vi "判断调焦 - 近.vi"(0 "Arr Refnum":refnum<vi>, 9 "选项":dbl min=0.0 max=5.0 step=1.0, 11 "error in":errorcluster) -> (4 "垂直清晰度-数值":dbl, 6 "垂直清晰度":bool, 8 "水平清晰度-数值":dbl, 10 "水平清晰度":bool, 15 "error out":errorcluster)   [LabVIEW 2016]
uses:
  <vilib>/Analysis/baseanly.llb/Mean (DBL).vi
  <vilib>/Analysis/NI_AALBase.lvlib
panel:
  out "Value":u16[][](array[numeric])
  out "Max value":dbl
  out "Min value":dbl
  out "Y坐标":dbl
  out "X 坐标":dbl
  out "垂直Bre":dbl
  out "水平Bre":dbl
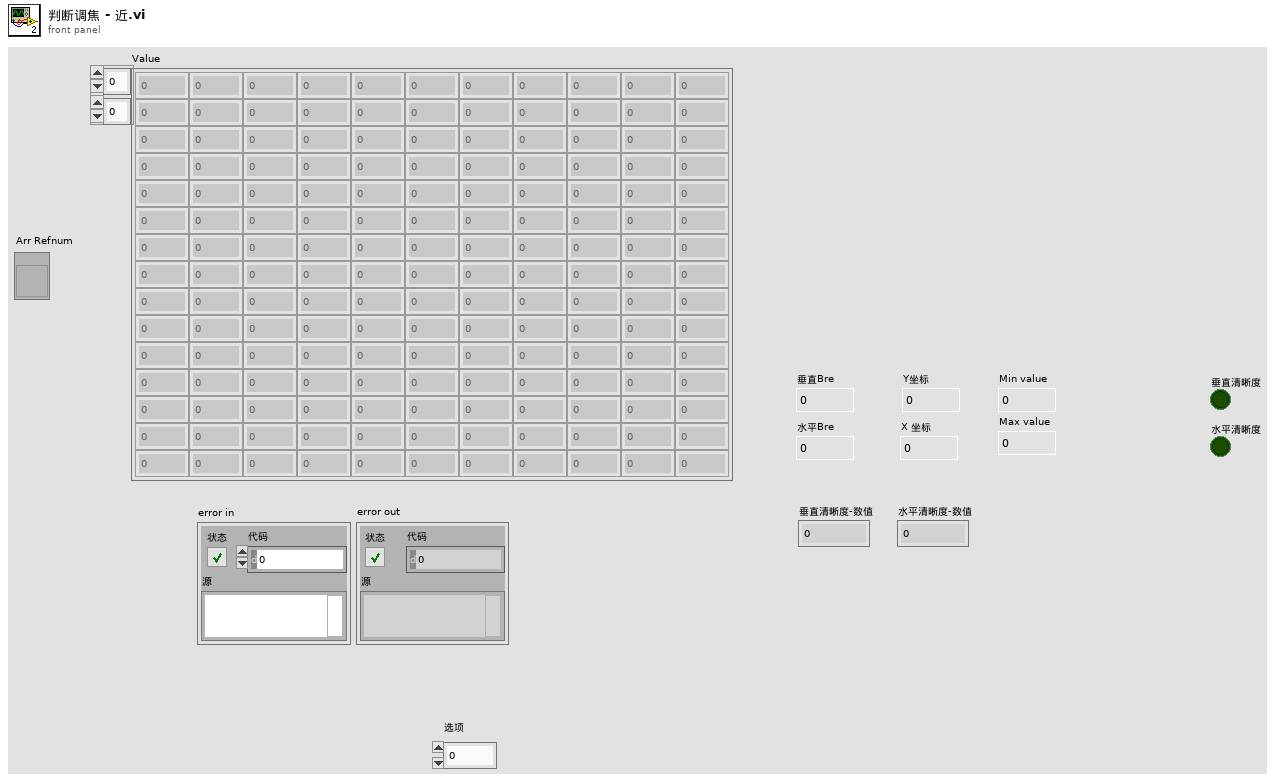
[diagram p1: front panel]
types:
  T1 = cluster{"CalData":path, "Datasave":path, "Data":path}
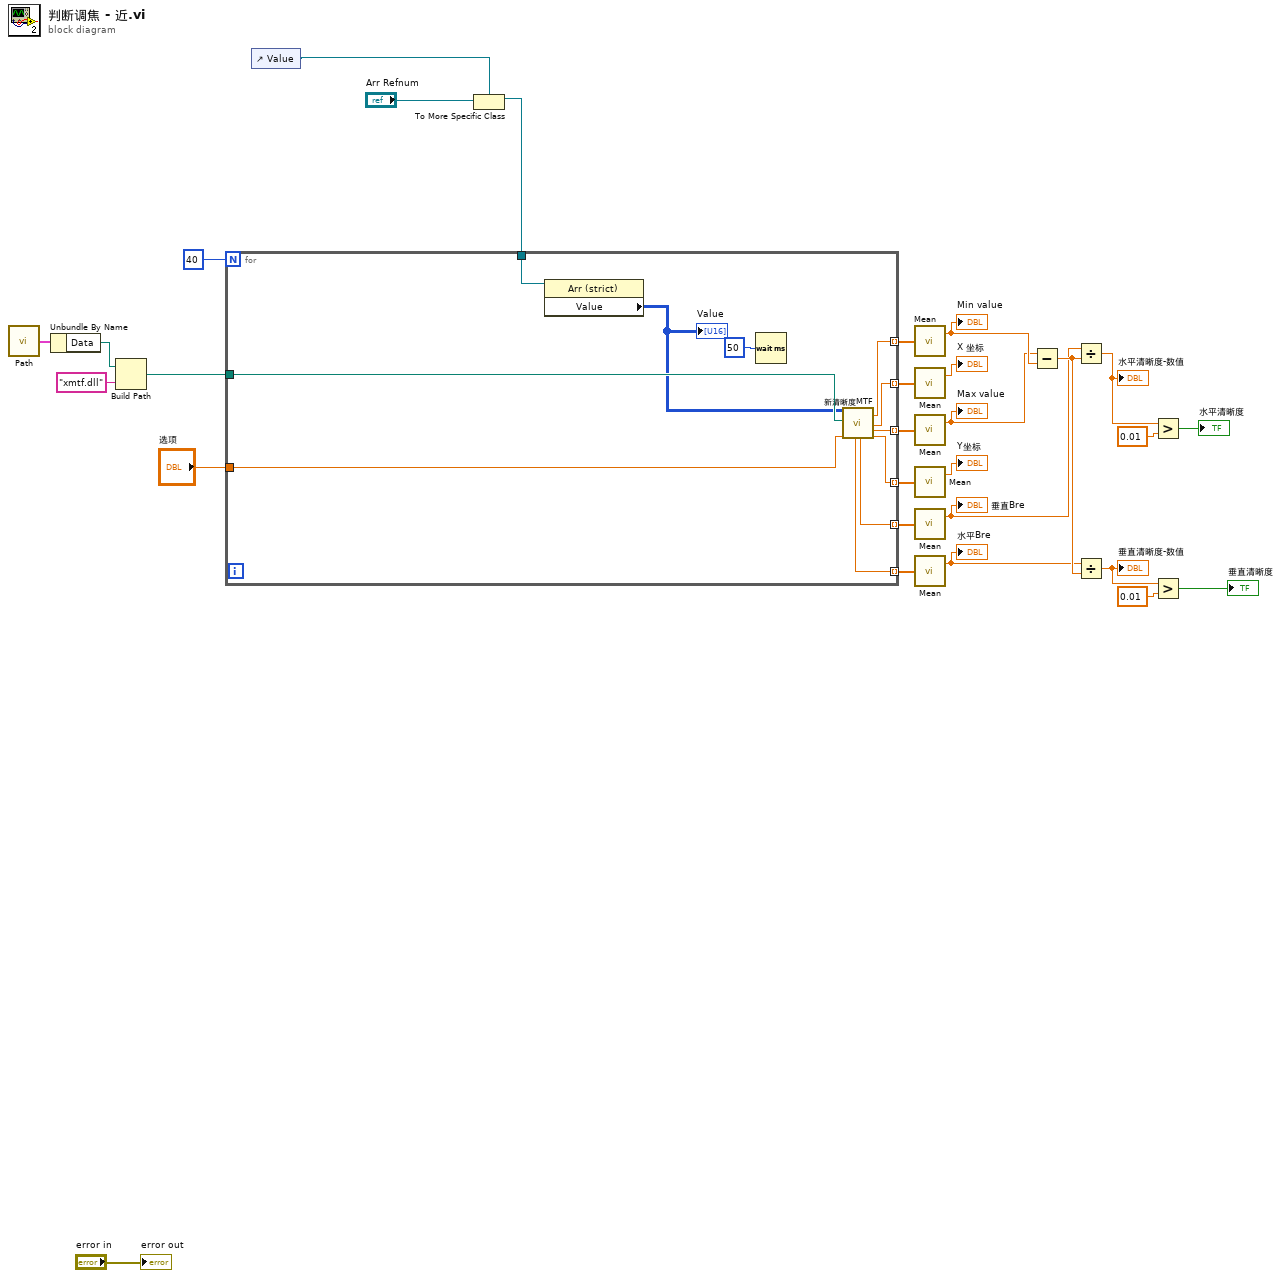
[diagram p0: block diagram]
diagram:
  n1 = call "Path.vi"() -> ("path"=w8:T1)  [unwired: 9 in]
  n2 = Unbundle By Name(w8) -> ("Data"=w6:path)
  n3 = Build Path(base path=w6, name or relative path="xmtf.dll") -> (appended path=w5:path)
  n4 = control-ref of="Value"() -> (w2:refnum<vi>)
  n5 = To More Specific Class(target class=w2, reference="Arr Refnum") -> (specific class reference=w3:refnum<vi>)  [unwired: 1 in, 1 out]
  n6 = for {
    N: 40 -> [_]
    tunnel: [w40] -> w9 mode=indexing
    tunnel: [w39] -> w14 mode=indexing
    tunnel: [w38] -> w18 mode=indexing
    tunnel: [w37] -> w12 mode=indexing
    tunnel: [w36] -> w15 mode=indexing
    tunnel: [w35] -> w19 mode=indexing
    tunnel: "选项" -> [w34]
    tunnel: w5 -> [w32]
    tunnel: w3 -> [w31]
    n7 = property class="Arr (strict)"(reference=w31) -> ("Value"=w30:u16[][])  [unwired: 1 in, 2 out]
    "Value" <- w30
    n8 = Wait (ms)(milliseconds to wait=u32 50) -> ()  [unwired: 1 out]
    n9 = call "新清晰度MTF.vi"("Image Pixels"=w30, "path in"=w32, "焦距选择"=w34) -> ("水平Bre"=w40:dbl, "垂直Bre"=w37:dbl, "Min value"=w38:dbl, "X 坐标"=w36:dbl, "Max value"=w39:dbl, "Y坐标"=w35:dbl)  [unwired: 9 in, 2 out]
  }
  n10 = call-poly <vilib>:"Mean.vi"("X"=w18) -> ("mean"=w17:dbl)  [unwired: 1 out]
  "Min value" <- w17
  n11 = call-poly <vilib>:"Mean.vi"("X"=w15) -> ("mean"=→"X 坐标":dbl)  [unwired: 1 out]
  n12 = call-poly <vilib>:"Mean.vi"("X"=w14) -> ("mean"=w13:dbl)  [unwired: 1 out]
  "Max value" <- w13
  n13 = call-poly <vilib>:"Mean.vi"("X"=w19) -> ("mean"=→"Y坐标":dbl)  [unwired: 1 out]
  n14 = call-poly <vilib>:"Mean.vi"("X"=w12) -> ("mean"=w11:dbl)  [unwired: 1 out]
  "垂直Bre" <- w11
  n15 = call-poly <vilib>:"Mean.vi"("X"=w9) -> ("mean"=w10:dbl)  [unwired: 1 out]
  "水平Bre" <- w10
  n16 = Subtract(x=w13, y=w17) -> (x-y=w24:dbl)
  n17 = Divide(x=w11, y=w24) -> (x/y=w23:dbl)
  "水平清晰度-数值" <- w23
  n18 = Divide(x=w10, y=w24) -> (x/y=w25:dbl)
  "垂直清晰度-数值" <- w25
  n19 = Greater?(x=w23, y=0.01) -> (0:→"水平清晰度":bool)
  n20 = Greater?(x=w25, y=0.01) -> (0:→"垂直清晰度":bool)
  "error out" <- "error in"
